vi "RSZVB Set Marker Search Result State.vi"(7 "Search Results (F: Off)":bool, 8 "error in (no error)":errorcluster {"code" format="%.0x"}, 9 "Marker (1)":i32=1, 10 "Channel (Trace) (1)":i32=1, 11 "VISA session":refnum<visa-resource-name>) -> (0 "error out":errorcluster {"code" format="%.0x"}, 3 "dup VISA session":refnum<visa-resource-name>)   [LabVIEW 2011]
doc: "This VI shows or hides the bandfilter search results in the diagram area.\n\nRemote-control command(s):\nCALCulate<Chn>:MARKer<Mk>:FUNCtion:EXECute BFILter\nCALCulate<Chn>:MARKer<Mk>:SEARch:BFILter:RESult[:STATe] <Boolean>"
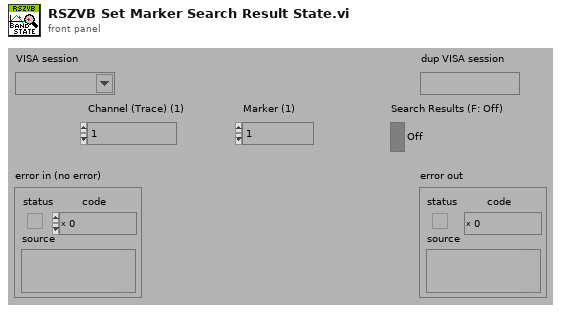
[diagram p1: front panel]
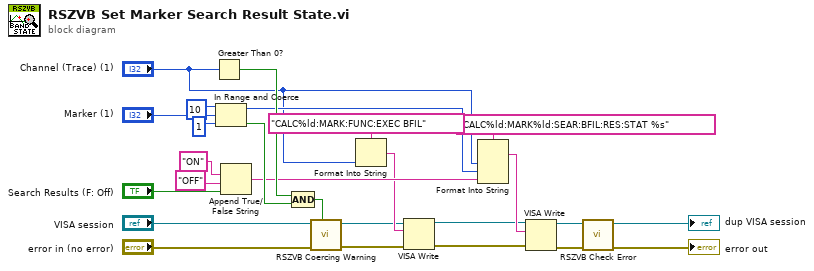
[diagram p0: block diagram]
diagram:
  n1 = Greater Than 0?(x="Channel (Trace) (1)") -> (x > 0?=w18:bool)
  n2 = In Range and Coerce(upper limit=10, x="Marker (1)", lower limit=1) -> (coerced(x)=w14:i32, In Range?=w16:bool)
  n3 = Append True/False String(1:"Search Results (F: Off)", 2:"OFF", 3:"ON") -> (0:w15:string)  [unwired: 1 in]
  n4 = Compound Arithmetic op=AND(w18, w16) -> (w17:bool)
  n5 = call "RSZVB Coercing Warning.vi"("In Range?"=w17, "error in (no error)"="error in (no error)", "VISA session"="VISA session") -> ("error out"=w3:errorcluster, "dup VISA session"=w4:refnum<visa-resource-name>)  [unwired: 7 in]
  n6 = Format Into String(format string="CALC%ld:MARK:FUNC:EXEC BFIL", "Channel (Trace) (1)") -> (resulting string=w6:string)  [unwired: 2 in, 1 out]
  n7 = VISA Write(VISA resource name=w4, write buffer=w6, error in (no error)=w3) -> (VISA resource name out=w2:refnum<visa-resource-name>, error out=w1:errorcluster)  [unwired: 1 out]
  n8 = Format Into String(format string="CALC%ld:MARK%ld:SEAR:BFIL:RES:STAT %s", "Channel (Trace) (1)", w14, w15) -> (resulting string=w23:string)  [unwired: 2 in, 1 out]
  n9 = VISA Write(VISA resource name=w2, write buffer=w23, error in (no error)=w1) -> (VISA resource name out=w24:refnum<visa-resource-name>, error out=w25:errorcluster)  [unwired: 1 out]
  n10 = call "RSZVB Check Error.vi"("error in (no error)"=w25, "VISA session"=w24) -> ("error out"=→"error out":errorcluster, "dup VISA session"=→"dup VISA session":refnum<visa-resource-name>)  [unwired: 8 in]
